vi "Set Inline Buffer.vi"(10 "Inline Buffer":refnum<class "Double Pointer.lvclass">, 11 "Transfer in":refnum<class "Transfer.lvclass">) -> (3 "Transfer out":refnum<class "Transfer.lvclass">)   [LabVIEW 2017, in "Data Sharing Framework Core.lvlib" / "Data Sharing Framework Engine.lvlib" / "Transfer.lvclass"]
uses:
  Transfer.lvclass
  Internal/Memory/Double Pointer/Double Pointer.lvclass
  Transfer.lvclass/Transfer.ctl
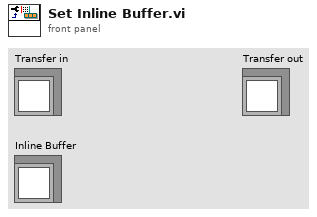
[diagram p1: front panel]
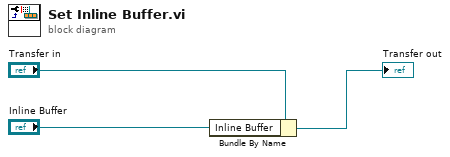
[diagram p0: block diagram]
diagram:
  n1 = Bundle By Name(cluster="Transfer in", "Inline Buffer"="Inline Buffer") -> (→"Transfer out":refnum<class "Transfer.lvclass">)
